vi "oax_gsLoad processed data with Dialog.vi"(6 "EXE distribution?":bool=TRUE, 8 "error in (not an error)":errorcluster, 10 "start path":path) -> (0 "error out":errorcluster, 1 "parameters":cluster{"sample rate":sgl, "pulses/rev":i32} {"sample rate" format="%.2f"}, 2 "speed profile":T2 {"speed [RPM]" format="%.2f"; "time [s]" format="%.2f"}, 3 "S&V samples":dbl[](array[numeric]) format="%.2f", 4 "window info":T1={"window type"=3, "window length"=2048} {"window type" items=["None"=0, "Hanning"=1, "Hamming"=2, "Blackman-Harris"=3, "Exact Blackman"=4, "Blackman"=5, "Flat Top"=6, "4 Term B-Harris"=7, "7 Term B-Harris"=8, "Low Sidelobe"=9, "Gaussian"=62]; "window length" min=0}, 5 "lables":cluster{"tach lable":string, "S&V lable":string}, 7 "file path out":path)   [LabVIEW 2017]
uses:
  <vilib>/addons/Sound and Vibration/Order Analysis/Tach Process/SubVIs/speed profile.ctl
  <vilib>/addons/Sound and Vibration/Order Analysis/Ref Gabor Order Tracking/window information.ctl
  <vilib>/addons/Sound and Vibration/Order Analysis/Gabor Order Tracking/SoundVib_Gabor.lvlib
  <vilib>/addons/Sound and Vibration/Order Analysis/Tach Process/SoundVib_TachProcess.lvlib
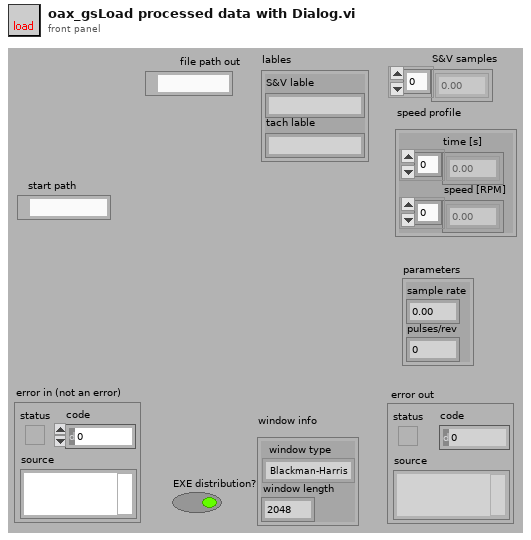
[diagram p1: front panel]
types:
  T1 = typedef "SoundVib_Gabor.lvlib/window information.ctl" = cluster{"window type":u32, "window length":i32}
  T2 = typedef "SoundVib_TachProcess.lvlib/speed profile.ctl" = cluster{"time [s]":dbl[], "speed [RPM]":dbl[]}
  T3 = cluster{"lables":cluster{"tach lable":string, "S&V lable":string}, "S&V samples":dbl[], "speed profile":cluster{"time [s]":dbl[], "speed [rpm]":dbl[]}, "parameters":cluster{"sample rate":sgl, "pulses/rev":i32}, "window info":cluster{"window type":enum32{"Hanning", "Hamming", "Blackman", "Gaussian"}, "window length":i32}}[]
  T4 = cluster{"lables":cluster{"tach lable":string, "S&V lable":string}, "S&V samples":dbl[], "speed profile":cluster{"time [s]":dbl[], "speed [rpm]":dbl[]}, "parameters":cluster{"sample rate":sgl, "pulses/rev":i32}, "window info":cluster{"window type":enum32{"Hanning", "Hamming", "Blackman", "Gaussian"}, "window length":i32}}
  T5 = cluster{"window type":enum32{"Hanning", "Hamming", "Blackman", "Gaussian"}, "window length":i32}
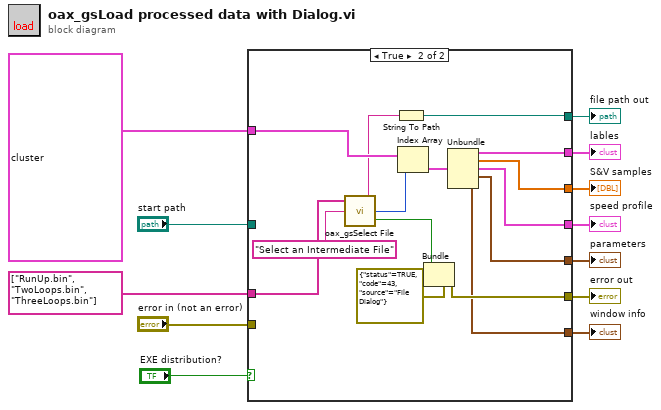
[diagram p0: block diagram]
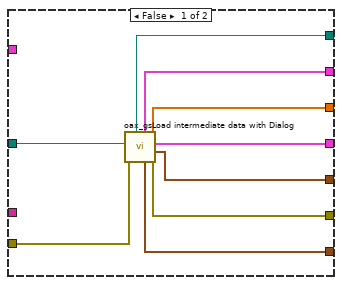
[diagram p2: hidden frame]
diagram:
  n1 = case shown="True" "EXE distribution?" {
    tunnel: [w21 w25] -> w12
    tunnel: [w20 w31] -> w11
    tunnel: [w19 w28] -> w10
    tunnel: [w18 w30] -> w9
    tunnel: [w17 w29] -> w8
    tunnel: [w16 w27] -> w7
    tunnel: [w15 w33] -> w6
    tunnel: "start path" -> [w14 _]
    tunnel: "error in (not an error)" -> [w13 _]
    tunnel: T3 [{"lables"={"tach lable"="tacho (V)", "S&V lable"="acc H (m/s^2)"}, "S&V samples"=array[55296 elements], "speed profile"={"time [s]"=array[1418 elements], "speed [rpm]"=array[1418 elements]}, "parameters"={"sample rate"=4000.0, "pulses/rev"=2}, "window info"={"window type"=enum."Gaussian", "window length"=2048}}, {"lables"={"tach lable"="Tach (V)", "S&V lable"="Acc Y (g)"}, "S&V samples"=array[73728 elements], "speed profile"={"time [s]"=array[1257 elements], "speed [rpm]"=array[1257 elements]}, "parameters"={"sample rate"=5000.0, "pulses/rev"=2}, "window info"={"window type"=enum."Gaussian", "window length"=2048}}, {"lables"={"tach lable"="Tach (V)", "S&V lable"="Acc X (g)"}, "S&V samples"=array[73728 elements], "speed profile"={"time [s]"=array[1212 elements], "speed [rpm]"=array[1212 elements]}, "parameters"={"sample rate"=5000.0, "pulses/rev"=2}, "window info"={"window type"=enum."Gaussian", "window length"=1024}}] ("Array") -> [_ w35]
    tunnel: string[] ["RunUp.bin", "TwoLoops.bin", "ThreeLoops.bin"] ("Item Names") -> [_ w23]
    frame False {
      n2 = call <vilib>:"oax_gsLoad intermediate data with Dialog.vi"("error in (not an error)"=w13, "start path"=w14) -> ("error out"=w15:errorcluster, "parameters"=w19:cluster{"sample rate":sgl, "pulses/rev":i32}, "speed profile"=w17:T2, "S&V samples"=w18:dbl[], "window info"=w16:T1, "lables"=w20:cluster{"tach lable":string, "S&V lable":string}, "file path out"=w21:path)  [unwired: 3 in]
    }
    frame True {
      n3 = call <vilib>:"oax_gsSelect File.vi"("prompt"="Select an Intermediate File", "file names"=w23) -> ("canceled"=w34:bool, "index"=w36:i32, "file name"=w26:string)  [unwired: 1 in]
      n4 = String To Path(string=w26) -> (path=w25:path)
      n5 = Index Array(array=w35, index=w36) -> (element=w32:T4)
      n6 = Bundle(cluster=errorcluster {"status"=TRUE, "code"=43, "source"="File Dialog"} ("error out"), "status"=w34) -> (w33:errorcluster)  [unwired: 2 in]
      n7 = Unbundle(w32) -> ("lables"=w31:cluster{"tach lable":string, "S&V lable":string}, "S&V samples"=w30:dbl[], "speed profile"=w29:cluster{"time [s]":dbl[], "speed [rpm]":dbl[]}, "parameters"=w28:cluster{"sample rate":sgl, "pulses/rev":i32}, "window info"=w27:T5)
    }
  }
  "S&V samples" <- w9
  "speed profile" <- w8
  "window info" <- w7
  "error out" <- w6
  "file path out" <- w12
  "parameters" <- w10
  "lables" <- w11
